vi "Untitled 1 (SubVI).vi"(11 "pieceOfWorld in":T2[][](array[typedef])) -> (1 "column":i32, 2 "row":i32, 3 "foodAmount":T1)   [LabVIEW 2015, in "PolyVIEW.lvclass"]
uses:
  PolyVIEW.lvclass
  actors/world/typedefs/worldCell_cluster.ctl
  actors/world/typedefs/markValue_cluster.ctl
  actors/world/typedefs/markValue.ctl
  actors/world/typedefs/markVolume.ctl
  actors/world/typedefs/amountOfFood.ctl
  actors/world/typedefs/anthillType_enum.ctl
  actors/world/world.lvlib
panel:
  out "found?":bool
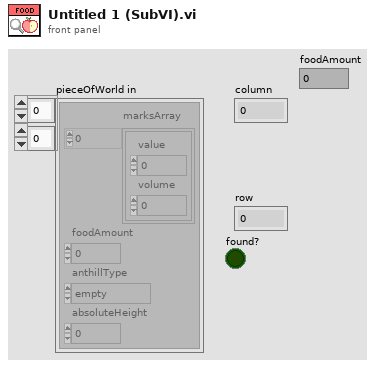
[diagram p1: front panel]
types:
  T1 = typedef "world.lvlib/amountOfFood.ctl" = i32
  T2 = typedef "world.lvlib/worldCell_cluster.ctl" = cluster{"marksArray":T3[], "foodAmount":T1, "anthillType":T6, "absoluteHeight":u8}
  T3 = typedef "world.lvlib/markValue_cluster.ctl" = cluster{"value":T4, "volume":T5}
  T4 = typedef "world.lvlib/markValue.ctl" = u8
  T5 = typedef "world.lvlib/markVolume.ctl" = u16
  T6 = typedef "world.lvlib/anthillType_enum.ctl" = enum16{"empty", "own", "rival"}
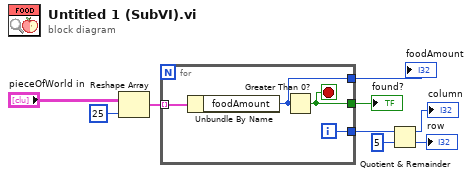
[diagram p0: block diagram]
diagram:
  n1 = Reshape Array("pieceOfWorld in", 25 ("dimension size")) -> (w7:T2[])
  n2 = for {
    tunnel: w7 -> [w13] mode=indexing
    tunnel: [w12] -> w2
    tunnel: [w11] -> w5
    tunnel: [w10] -> w1
    i -> [w12]
    stop <- w11 stop-if-true
    n3 = Unbundle By Name(w13) -> ("foodAmount"=w10:T1)
    n4 = Greater Than 0?(x=w10) -> (x > 0?=w11:bool)
  }
  "found?" <- w5
  "foodAmount" <- w1
  n5 = Quotient & Remainder(x=w2, y=5) -> (x-y*floor(x/y)=→"column":i32, floor(x/y)=→"row":i32)
